vi "Launch Local Reconfig.vi"(8 "error in (no error)":errorcluster, 10 "Config Channels":dbl[](array[numeric]), 11 "Local Reconfig VI Ref":refnum<vi>) -> (0 "error out":errorcluster)   [LabVIEW 2016, in "Scan Engine Custom Device.lvlib"]
uses:
  Scan Engine Custom Device.lvlib
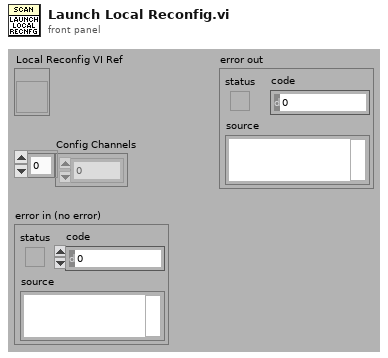
[diagram p1: front panel]
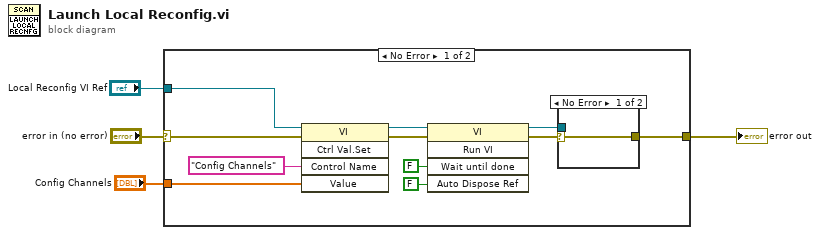
[diagram p0: block diagram]
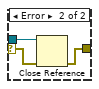
[diagram p2: hidden frame]
diagram:
  n1 = case shown="No Error" "error in (no error)" {
    selector: "error in (no error)" -> [w5 w20]
    tunnel: "Config Channels" -> [w15 _]
    tunnel: "Local Reconfig VI Ref" -> [w12 _]
    tunnel: [w10 w20] -> w2
    frame No Error {
      n2 = invoke class="VI" method="Ctrl Val.Set"(reference=w12, error in=w5, "Control Name"="Config Channels", "Value"=w15) -> (reference out=w13:refnum<vi>, error out=w14:errorcluster)  [unwired: 1 in, 3 out]
      n3 = invoke class="VI" method="Run VI"(reference=w13, error in=w14, "Wait until done"=FALSE ("Wait Until Done"), "Auto Dispose Ref"=FALSE ("Auto Dispose Reference")) -> (reference out=w6:refnum<vi>, error out=w7:errorcluster)  [unwired: 1 in, 3 out]
      n4 = case shown="No Error" w7 {
        selector: w7 -> [w16 w18]
        tunnel: w6 -> [_ w19]
        tunnel: [w16 w17] -> w10
        frame No Error {
        }
        frame Error {
          n5 = Close Reference(reference=w19, error in (no error)=w18) -> (error out=w17:errorcluster)
        }
      }
    }
    frame Error {
    }
  }
  "error out" <- w2
